vi "Average.vi"(1 "z":dbl, 2 "x":dbl) -> (0 "y":dbl)   [LabVIEW 2012]
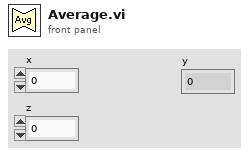
[diagram p1: front panel]
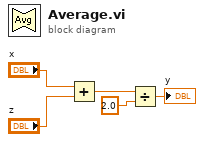
[diagram p0: block diagram]
diagram:
  n1 = Add(x="x", y="z") -> (x+y=w2:dbl)
  n2 = Divide(x=w2, y=2.0) -> (x/y=→"y":dbl)
